vi "check_option.vi"(7 "Attribute":T1={"Identifier"="", "Descriptive name"="", "Data Type"=enum."Integer 32", "Command"="", "Access"=2, "Range Table"="", "Read Callback"="", "Write Callback"="", "Range Callback"="", "Check Callback"="", "Rngtable Callback"="", "Coerce Callback"="", "Supported Models"="", "Instrument Options"="", "Repeated Capabilities"="", "Check Status Callback"="", "Index"=0, "Flag: OPC Wait"=FALSE, "Flag: Dont check status"=FALSE, "Flag: Cache Only"=FALSE} {"Access" items=["Read Only", "Write Only", "Read/Write"]}, 8 "error in":errorcluster, 11 "VISA resource name":refnum<visa-resource-name>) -> (0 "error out":errorcluster, 3 "VISA resource name out":refnum<visa-resource-name>)   [LabVIEW 2014, in "rszvl_rsidr_core.lvlib"]
uses:
  rszvl_rsidr_core.lvlib
  type_Attribute.ctl
  type_Attribute_Data_Type.ctl
  type_Error_Codes.ctl
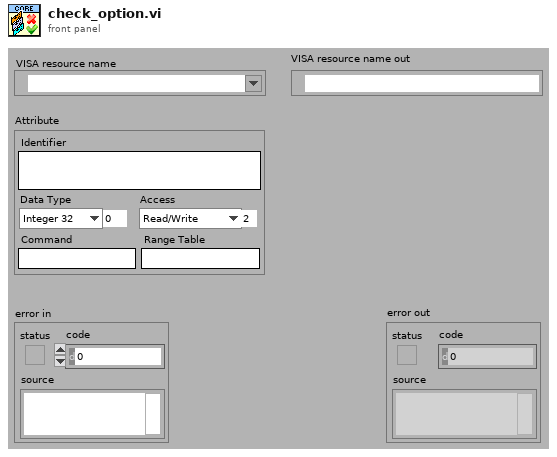
[diagram p1: front panel]
types:
  T1 = typedef "rszvl_rsidr_core.lvlib/type_Attribute.ctl" = cluster{"Identifier":string, "Descriptive name":string, "Data Type":T2, "Command":string, "Access":u16, "Range Table":string, "Read Callback":string, "Write Callback":string, "Range Callback":string, "Check Callback":string, "Rngtable Callback":string, "Coerce Callback":string, "Supported Models":string, "Instrument Options":string, "Repeated Capabilities":string, "Check Status Callback":string, "Index":i32, "Flag: OPC Wait":bool, "Flag: Dont check status":bool, "Flag: Cache Only":bool}
  T2 = typedef "rszvl_rsidr_core.lvlib/type_Attribute_Data_Type.ctl" = enum16{"Integer 32", "Double", "String", "Boolean", "None", "Integer 64"}
  T3 = typedef "rszvl_rsidr_core.lvlib/type_Error_Codes.ctl" = enum16{"No_error", "VISA_err_ResourceNotFound", "VISA_err_Timeout", "VISA_warn_MoreDataAvailable", "RS_err_MissingCallback", "RS_err_InvalidAttribute", "RS_err_InvalidValue", "RS_err_UnknownResource", "RS_err_AlreadyInitialized", "RS_err_InstrumentStatus", "RS_err_BadRepCapName", "RS_err_TypesMismatch", "RS_err_ValueNotSupported", "RS_err_InvalidRngTable", "RS_err_IDqueryFail", "RS_err_UnexpResponse", "VISA_warn_ConfigNotLoaded", "RS_err_AttributeNotReadable", "RS_err_AttributeNotWritable", "RS_err_InstrumentType", "RS_err_InstrumentOption", "VISA_err_InvalidSize", "RS_err_ReliabilityIndicator", "VISA_warn_UnknownStatus", "VISA_warn_TermCharRead", "VISA_err_IO_error"}
  T4 = typedef "rszvl_rsidr_core.lvlib/type_Session_Data.ctl" = cluster{"Instr type":string, "Instr type for err. msg.":string, "Installed Options":string[], "OPC Timeout":i32, "Query Instrument Status":bool, "Check Range":bool, "Check Options":bool, "Add LF to Write":bool, "Simulate":bool, "Logging":bool, "Logging params":variant, "Interface Type":enum16{"Unknown", "GPIB", "VXI", "GPIB_VXI", "ASRL", "PXI", "TCPIP", "USB", "SOCKET"}, "Fast Sweep":i32, "AdditionalFlags":i32, "WaitBeforeWrite":i32, "WaitBeforeRead":i32, "BinDataChunkSize":i64}
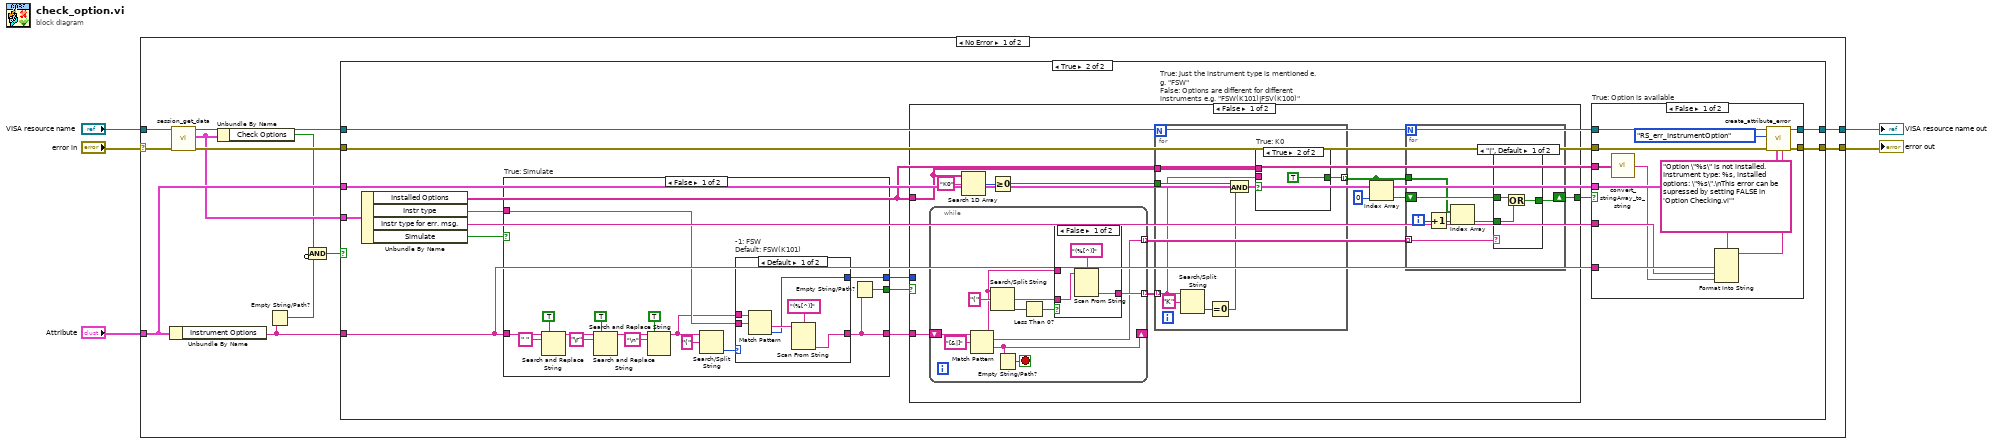
[diagram p0: block diagram]
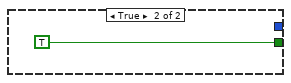
[diagram p4: hidden frame]
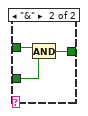
[diagram p5: hidden frame]
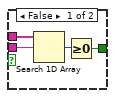
[diagram p6: hidden frame]
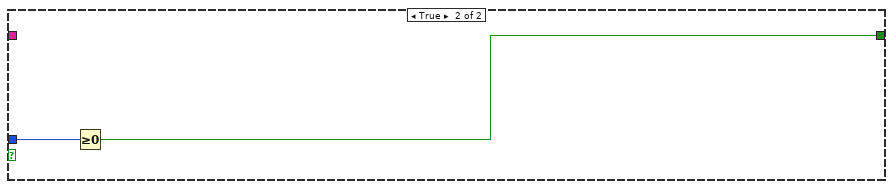
[diagram p8: hidden frame]
diagram:
  n1 = case shown="No Error" "error in" {
    selector: "error in" -> [w12 w127]
    tunnel: [w17 w127] -> w5
    tunnel: "Attribute" -> [w16 _]
    tunnel: "VISA resource name" -> [w13 w128]
    tunnel: [w14 w128] -> w2
    frame No Error {
      n2 = Unbundle By Name(w16) -> ("Instrument Options"=w15:string)
      n3 = call "session_get_data.vi"("error in"=w12, "VISA resource name"=w13) -> ("error out"=w10:errorcluster, "Session User Data out"=w9:T4, "VISA resource name out"=w11:refnum<visa-resource-name>)  [unwired: 7 in]
      n4 = Unbundle By Name(w9) -> ("Check Options"=w8:bool)
      n5 = Empty String/Path?(string/path=w15) -> (empty?=w7:bool)
      n6 = Compound Arithmetic op=AND(w8, invert w7) -> (w6:bool)
      n7 = case shown="True" w6 {
        tunnel: w10 -> [w19 w24]
        tunnel: [w19 w33] -> w17
        tunnel: w15 -> [_ w30]
        tunnel: w16 -> [_ w31]
        tunnel: w11 -> [w18 w23]
        tunnel: [w18 w22] -> w14
        tunnel: w9 -> [_ w25]
        frame False {
        }
        frame True {
          n8 = Unbundle By Name(w25) -> ("Installed Options"=w21:string[], "Instr type"=w32:string, "Instr type for err. msg."=w29:string, "Simulate"=w20:bool)
          n9 = case "True: Simulate" shown="False" w20 {
            tunnel: w32 -> [w50 _]
            tunnel: w30 -> [w49 _]
            tunnel: [w37 _] -> w28
            tunnel: [w35 TRUE] -> w27
            tunnel: [w36 _] -> w26
            frame False {
              n10 = Search and Replace String(replace all?=TRUE ("replace all? (F)"), input string=w49, search string=" ") -> (result string=w42:string)  [unwired: 5 in, 3 out]
              n11 = Search and Replace String(replace all?=TRUE ("replace all? (F)"), input string=w42, search string="\r") -> (result string=w41:string)  [unwired: 5 in, 3 out]
              n12 = Search and Replace String(replace all?=TRUE ("replace all? (F)"), input string=w41, search string="\n") -> (result string=w38:string)  [unwired: 5 in, 3 out]
              n13 = Search/Split String(string=w38, search string/char (-)="(") -> (offset of match=w39:i32)  [unwired: 1 in, 2 out]
              n14 = case "-1: FSW\nDefault: FSW(K101)" shown="Default" w39 {
                tunnel: w38 -> [w56 w57]
                tunnel: [w52 w57] -> w36
                tunnel: w50 -> [w55 _]
                tunnel: [w51 _] -> w37
                frame Default {
                  n15 = Match Pattern(string=w56, regular expression=w55) -> (after substring=w54:string, offset past match=w51:i32)  [unwired: 1 in, 2 out]
                  n16 = Scan From String(format string="(%[^)]", input string=w54) -> (output 1=w52:string)  [unwired: 3 in, 3 out]
                }
                frame -1 {
                }
              }
              n17 = Empty String/Path?(string/path=w36) -> (empty?=w35:bool)
            }
            frame True {
            }
          }
          n18 = case "True: Just the instrument type is mentioned e.g. \"FSW\"\nFalse: Options are different for different instruments e.g. \"FSW(K101)|FSV(K100)\"" shown="False" w27 {
            tunnel: [w66 w111] -> w34
            tunnel: w26 -> [w65 _]
            tunnel: w21 -> [w63 _]
            tunnel: w28 -> [_ w112]
            frame False {
              n19 = while {
                shift-right: [w96] -> _
                shift-left: w65 -> [w106]
                tunnel: [w99] -> w59 mode=indexing
                tunnel: [w98] -> w69 mode=indexing
                stop <- w104 stop-if-true
                n20 = Match Pattern(string=w106, regular expression="[&|]") -> (before substring=w97:string, match substring=w98:string, after substring=w96:string)  [unwired: 1 in, 1 out]
                n21 = Search/Split String(string=w97, search string/char (-)="(") -> (match + rest of string=w102:string, offset of match=w101:i32)  [unwired: 1 in, 1 out]
                n22 = Empty String/Path?(string/path=w96) -> (empty?=w104:bool)
                n23 = Less Than 0?(x=w101) -> (x < 0?=w100:bool)
                n24 = case shown="False" w100 {
                  tunnel: w102 -> [w107 _]
                  tunnel: [w108 w110] -> w99
                  tunnel: w97 -> [_ w110]
                  frame False {
                    n25 = Scan From String(format string="(%[^)]", input string=w107) -> (output 1=w108:string)  [unwired: 3 in, 3 out]
                  }
                  frame True {
                  }
                }
              }
              n26 = Search 1D Array(1D array=w63, element="K0") -> (index of element=w61:i32)  [unwired: 1 in]
              n27 = Greater Or Equal To 0?(x=w61) -> (x >= 0?=w60:bool)
              n28 = for {
                tunnel: w63 -> [w90]
                tunnel: [w89] -> w64 mode=indexing
                tunnel: w60 -> [w85]
                tunnel: w59 -> [w84] mode=indexing
                n29 = Search/Split String(string=w84, search string/char (-)="K") -> (offset of match=w87:i32)  [unwired: 1 in, 2 out]
                n30 = Equal To 0?(x=w87) -> (x = 0?=w86:bool)
                n31 = Compound Arithmetic op=AND(w85, w86) -> (w83:bool)
                n32 = case "True: K0" shown="True" w83 {
                  tunnel: w90 -> [w94 _]
                  tunnel: [w92 TRUE] -> w89
                  tunnel: w84 -> [w91 _]
                  frame False {
                    n33 = Search 1D Array(1D array=w94, element=w91) -> (index of element=w93:i32)  [unwired: 1 in]
                    n34 = Greater Or Equal To 0?(x=w93) -> (x >= 0?=w92:bool)
                  }
                  frame True {
                  }
                }
              }
              n35 = Index Array(array=w64, index=0) -> (element=w68:bool)
              n36 = for {
                tunnel: w69 -> [w70] mode=indexing
                tunnel: w64 -> [w74]
                shift-right: [w75] -> w66
                shift-left: w68 -> [w76]
                i -> [w72]
                n37 = Increment(x=w72) -> (x+1=w73:i32)
                n38 = Index Array(array=w74, index=w73) -> (element=w71:bool)
                n39 = case shown="\"|\", Default" w70 {
                  tunnel: w76 -> [w78 w82]
                  tunnel: [w79 w81] -> w75
                  tunnel: w71 -> [w77 w80]
                  frame "|", Default {
                    n40 = Or(x=w78, y=w77) -> (x .or. y?=w79:bool)
                  }
                  frame "&" {
                    n41 = And(x=w82, y=w80) -> (x .and. y?=w81:bool)
                  }
                }
              }
            }
            frame True {
              n42 = Greater Or Equal To 0?(x=w112) -> (x >= 0?=w111:bool)
            }
          }
          n43 = case "True: Option is available" shown="False" w34 {
            tunnel: w24 -> [w123 w126]
            tunnel: [w124 w126] -> w33
            tunnel: w31 -> [w120 _]
            tunnel: w30 -> [w122 _]
            tunnel: w29 -> [w114 _]
            tunnel: w23 -> [w117 w125]
            tunnel: [w116 w125] -> w22
            tunnel: w21 -> [w115 _]
            frame False {
              n44 = call "convert_stringArray_to_string.vi"("string array in"=w115) -> ("string out"=w113:string)  [unwired: 4 in]
              n45 = Format Into String(format string="Option \"%s\" is not installed. Instrument type: %s, installed options: \"%s\".\nThis error can be supressed by setting FALSE in 'Option Checking.vi'" ("string"), w122, w114, w113) -> (resulting string=w119:string)  [unwired: 2 in, 1 out]
              n46 = call "create_attribute_error.vi"("Error Elaboration (\"\")"=w119, "Attribute"=w120, "error in"=w123, "Error Enum in"=type_Error_Codes."RS_err_InstrumentOption" ("Error Enum in (from err to recompose)"), "VISA resource name"=w117) -> ("error out"=w124:errorcluster, "VISA resource name out"=w116:refnum<visa-resource-name>)  [unwired: 5 in]
            }
            frame True {
            }
          }
        }
      }
    }
    frame Error {
    }
  }
  "error out" <- w5
  "VISA resource name out" <- w2
